vi "Elapsed Time.vi"(11 "Mode 2":enum8{"Tele-Op", "Auto", ""}(ring)=enum."") -> (3 "Elapsed Time":dbl)   [LabVIEW 2011]
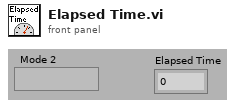
[diagram p1: front panel]
types:
  T1 = cluster{"Mode 2":enum8{"Tele-Op", "Auto", ""}, "millisecond timer value":u32}
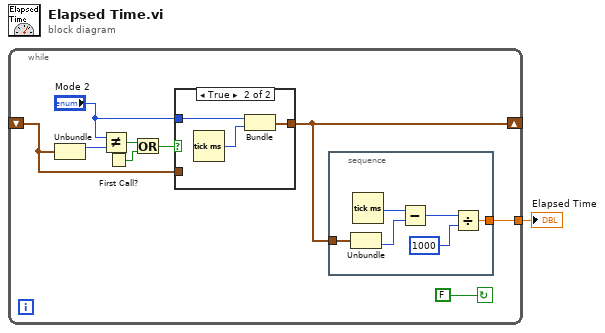
[diagram p0: block diagram]
diagram:
  n1 = while {
    shift-right: [w7] -> _
    shift-left: _ -> [w8]
    tunnel: [w6] -> w1
    stop <- FALSE continue-if-true
    n2 = Unbundle(w8) -> ("Mode 2"=w10:enum8{"Tele-Op", "Auto", ""})  [unwired: 1 out]
    n3 = Not Equal?(x="Mode 2", y=w10) -> (x != y?=w4:bool)
    n4 = First Call?() -> (First Call?: T/F=w3:bool)
    n5 = Or(x=w4, y=w3) -> (x .or. y?=w2:bool)
    n6 = case shown="True" w2 {
      tunnel: "Mode 2" -> [_ w20]
      tunnel: [w17 w18] -> w7
      tunnel: w8 -> [w17 _]
      frame False {
      }
      frame True {
        n7 = Tick Count (ms)() -> (millisecond timer value=w19:u32)
        n8 = Bundle("Mode 2"=w20, "millisecond timer value"=w19) -> (w18:T1)  [unwired: 1 out]
      }
    }
    n9 = stacked-sequence {
      tunnel: w7 -> [w13]
      tunnel: [w11] -> w6
      frame #0 {
        n10 = Unbundle(w13) -> ("millisecond timer value"=w12:u32)  [unwired: 1 out]
        n11 = Tick Count (ms)() -> (millisecond timer value=w16:u32)
        n12 = Subtract(x=w16, y=w12) -> (x-y=w15:u32)
        n13 = Divide(x=w15, y=1000) -> (x/y=w11:dbl)
      }
    }
  }
  "Elapsed Time" <- w1
